vi "Array Summation.vi"(10 "Array - Numeric":dbl[](array[numeric])) -> (2 "Summation":dbl)   [LabVIEW 2015]
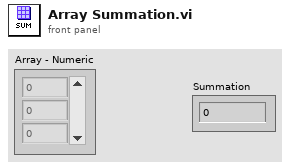
[diagram p1: front panel]
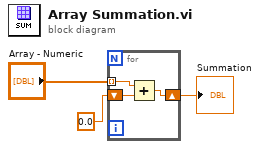
[diagram p0: block diagram]
diagram:
  n1 = for {
    tunnel: "Array - Numeric" -> [w6] mode=indexing
    shift-right: [w4] -> w1
    shift-left: 0.0 -> [w5]
    n2 = Add(x=w6, y=w5) -> (x+y=w4:dbl)
  }
  "Summation" <- w1
